vi "PS35_GetMoveState.vi"(3 "error in (no error)":errorcluster, 4 "Axis number":i32=1 min=0 max=3, 5 "Control unit ID":i32=1 min=1 max=10) -> (0 "error out":errorcluster, 1 "Move state":i32)   [LabVIEW 2020]
doc: "PS35_GetMoveState.vi, created: 04.03.2009 alex; last change: 22.10.2019 alex;\n\n<B>FUNCTION:</B> \n\nRead move state.\n----------------------------------------------------------------------------------------\n<B>INPUT:</B>\n[I32] <B>Control unit ID:</B> control unit index. (Default=1, Range=1...10) \n[I32] <B>Axis number:</B> axis number. (Default=1, Range=0...3)\n0 - read state of all axes,\n1...3 - read state of an axis. \n[CLU] <B>error in</B>\n----------------------------------------------------------------------------------------\n<B>OUTPUT:</B>\n[I32] <B>Move state:</B> state of an axis or all axes.\nAxis number = 0 (all axes)\n0 - all axes stand still and joystick mode is not active,\n1 - any axis runs or works in joystick mode.\nAxis number = 1...3 (an axis)\n0 - axis stands still,\n1 - axis runs in trapezoidal profile,\n2 - axis runs in S-curve profile,\n3 - axis runs to reference position,\n4 - axis releases active limit switches,\n5 - axis works in velocity mode,\n6 - axis works in joystick mode,\n7 - axis runs in trapezoidal profile with WMS (way measuring system),\n8 - axis runs in S-curve profile with WMS,\n9 - axis works in velocity mode with WMS,\n10 - axis works in velocity mode with continuous-path control.\n[CLU] <B>error out</B>\n----------------------------------------------------------------------------------------\n<B>SUB-VIs:</B>\nPS35_GetReadError.vi\n----------------------------------------------------------------------------------------\n<B>EXT-Calls:</B>\nps35.dll (V2.01)\n----------------------------------------------------------------------------------------"
uses:
  ps35.dll
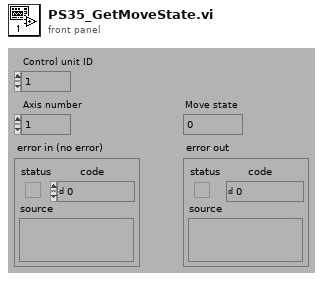
[diagram p1: front panel]
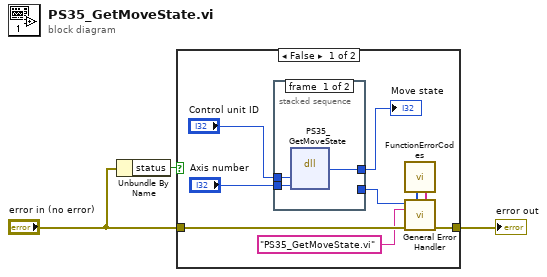
[diagram p0: block diagram]
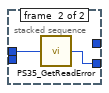
[diagram p2: hidden frame]
diagram:
  n1 = Unbundle By Name("error in (no error)") -> ("status"=w1:bool)
  n2 = case shown="False" w1 {
    tunnel: "error in (no error)" -> [w11 w18]
    tunnel: [w10 w18] -> w3
    frame False {
      n3 = stacked-sequence {
        tunnel: "Control unit ID" -> [w15 w17]
        tunnel: [w14 _] -> w9
        tunnel: [_ w16] -> w8
        tunnel: "Axis number" -> [w13 _]
        frame #0 {
          n4 = dll-call lib="C:/GEECS/Developers Version/source/Device Drivers/OwiSoft_PS35/OWISoftOEM/ps35/labview/lv82/ps35.dll" fn="PS35_GetMoveState" label="PS35_Get\nMoveState"("Index"=w15, "AxisNr"=w13) -> ("Rückgabetyp"=w14:i32)  [unwired: 5 in, 2 out]
        }
        frame #1 {
          n5 = call "PS35_GetReadError.vi"("Control unit ID"=w17) -> ("Read error"=w16:i32)
        }
      }
      "Move state" <- w9
      n6 = call "FunctionErrorCodes.vi"() -> ("[user-defined codes]"=w5:i32[], "[user-defined descriptions]"=w4:string[])  [unwired: 8 in]
      n7 = call "General Error Handler.vi"("[error code] (0)"=w8, "[user-defined codes]"=w5, "[user-defined descriptions]"=w4, "[error source] (\" \")"="PS35_GetMoveState.vi" ("[error source] (\" \")"), "error in (no error)"=w11) -> ("error out"=w10:errorcluster)  [unwired: 6 in, 4 out]
    }
    frame True {
    }
  }
  "error out" <- w3
